vi "SetParam.vi"(8 "error in":errorcluster caption="entrée d'erreur", 10 "fetch_lfw_people":T1={"funneled"=TRUE, "resize"=0.5, "min_faces_per_person"=0, "color"=FALSE, "slice_"={"Cluster"={"height"=70, "width"=195}, "Cluster 2"={"height"=78, "width"=172}}, "download_if_missing"=TRUE, "Returns"="Data"}, 11 "lfw_people.lvclass":refnum<class "lfw_people.lvclass">) -> (0 "error out":errorcluster caption="sortie d'erreur", 3 "lfw_people.lvclass":refnum<class "lfw_people.lvclass">)   [LabVIEW 2020, in "lfw_people.lvclass"]
doc: "Set Parameters"
uses:
  lfw_people.lvclass
  lfw_people.lvclass/lfw_people.ctl
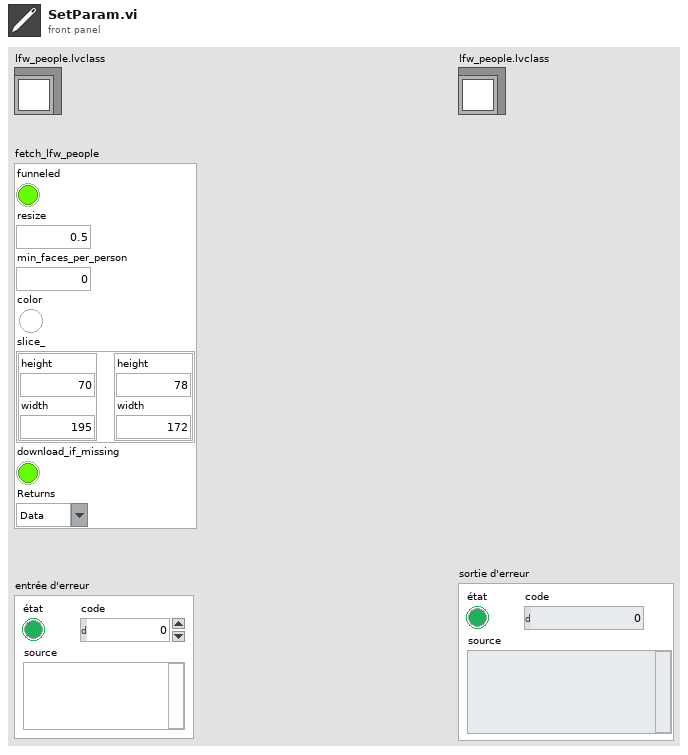
[diagram p1: front panel]
types:
  T1 = cluster{"funneled":bool, "resize":dbl, "min_faces_per_person":i32, "color":bool, "slice_":cluster{"Cluster":cluster{"height":u32, "width":u32}, "Cluster 2":cluster{"height":u32, "width":u32}}, "download_if_missing":bool, "Returns":string}
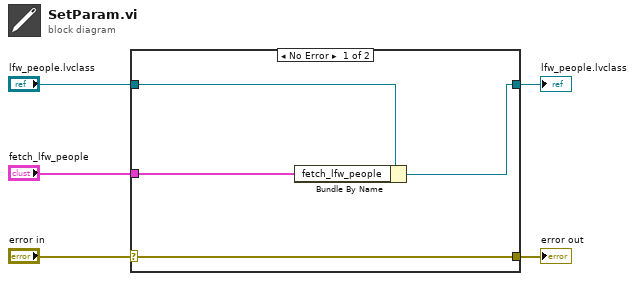
[diagram p0: block diagram]
diagram:
  n1 = case shown="No Error" "error in" {
    selector: "error in" -> [w9 w10]
    tunnel: [w9 w10] -> w4
    tunnel: [w7 w11] -> w2
    tunnel: "lfw_people.lvclass" -> [w8 w11]
    tunnel: "fetch_lfw_people" -> [w6 _]
    frame No Error {
      n2 = Bundle By Name(cluster=w8, "fetch_lfw_people"=w6) -> (w7:refnum<class "lfw_people.lvclass">)
    }
    frame Error {
    }
  }
  "error out" <- w4
  "lfw_people.lvclass" <- w2
